vi "setDevice.vi"(8 "error in (no error)":errorcluster, 10 "Device.lvclass":refnum<class "Device.lvclass">, 11 "AdvancedRemote in":refnum<class "AdvancedRemote.lvclass">) -> (0 "error out":errorcluster, 3 "AdvancedRemote out":refnum<class "AdvancedRemote.lvclass">)   [LabVIEW 2017, in "AdvancedRemote.lvclass"]
uses:
  AdvancedRemote.lvclass
  Device Class/Device.lvclass
  AdvancedRemote.lvclass/AdvancedRemote.ctl
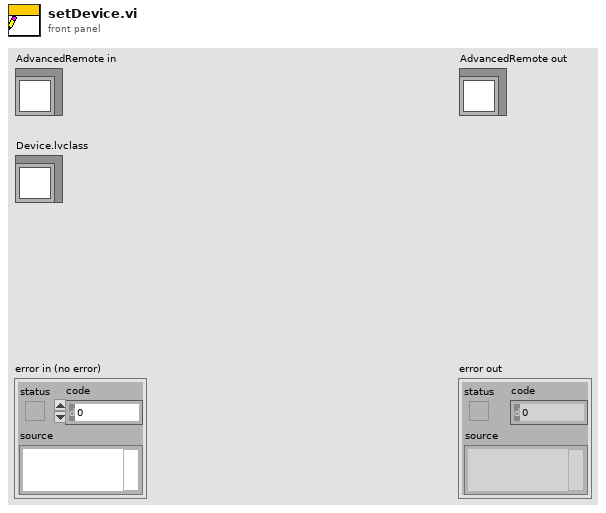
[diagram p1: front panel]
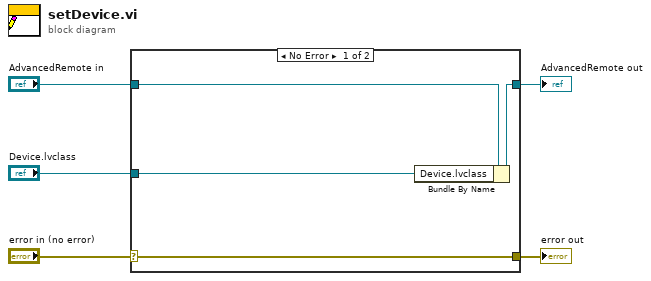
[diagram p0: block diagram]
diagram:
  n1 = case shown="No Error" "error in (no error)" {
    selector: "error in (no error)" -> [w9 w10]
    tunnel: [w9 w10] -> w4
    tunnel: [w7 w11] -> w2
    tunnel: "AdvancedRemote in" -> [w8 w11]
    tunnel: "Device.lvclass" -> [w6 _]
    frame No Error {
      n2 = Bundle By Name(cluster=w8, "Device.lvclass"=w6) -> (w7:refnum<class "AdvancedRemote.lvclass">)
    }
    frame Error {
    }
  }
  "error out" <- w4
  "AdvancedRemote out" <- w2
